vi "Scalar Charact Type.vi"() -> (0 "Charact Type":string)   [LabVIEW 2023, in "RFFixtureCharact.RFPM.lvlib" / "Scalar Charact Result Accessor.lvclass"]
uses:
  Scalar Charact Result Accessor.lvclass
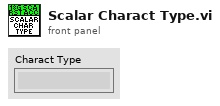
[diagram p1: front panel]
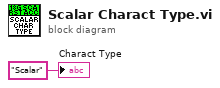
[diagram p0: block diagram]
diagram:
  "Charact Type" <- "Scalar"
